vi "PWRClose.vi"(8 "error in (no error)":errorcluster {"code" format="%.0x"}, 11 "PWR In":refnum<visa-resource-name>) -> (0 "error out":errorcluster)   [LabVIEW 2015]
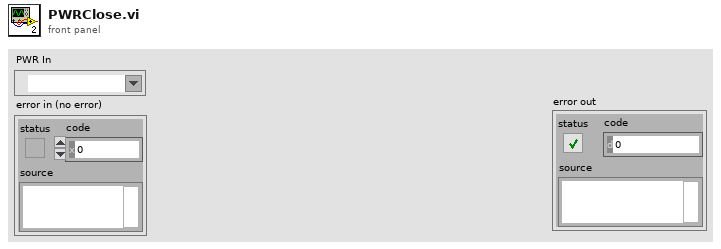
[diagram p1: front panel]
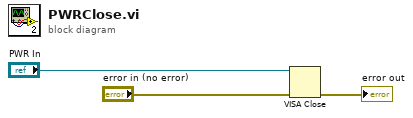
[diagram p0: block diagram]
diagram:
  n1 = VISA Close(VISA resource name="PWR In", error in (no error)="error in (no error)") -> (error out=→"error out":errorcluster)
